vi "Make.vi"(8 "error in (no error)":errorcluster, 10 "Actor":string) -> (0 "error out":errorcluster, 3 "Test-Client out":refnum<class "Test-Client.lvclass">)   [LabVIEW 2020, in "Test-Client.lvlib" / "Test-Client.lvclass"]
uses:
  Test-Client.lvclass
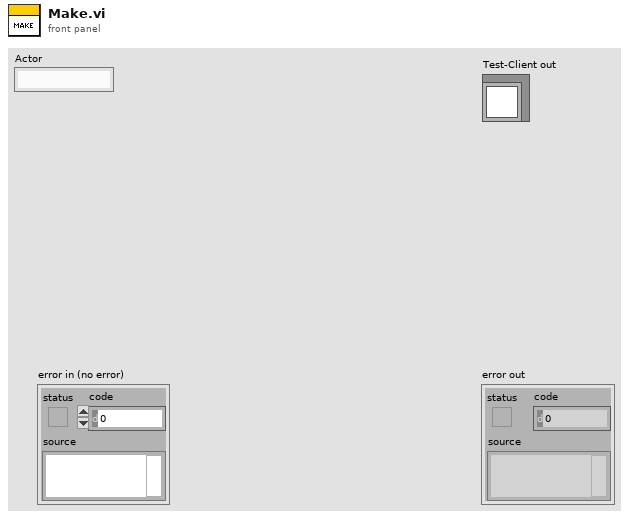
[diagram p1: front panel]
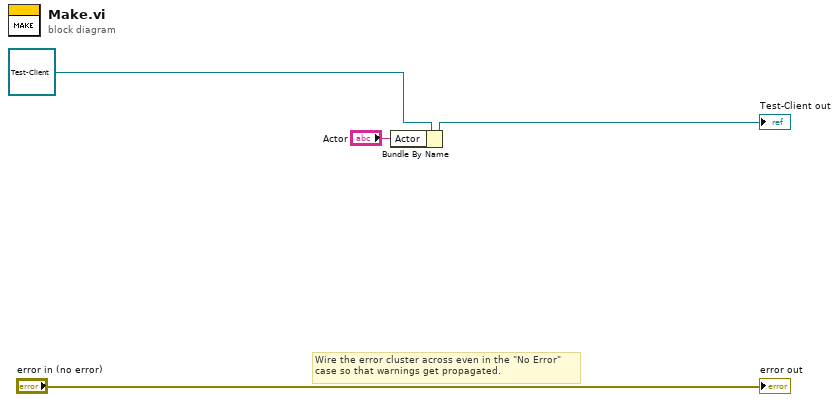
[diagram p0: block diagram]
diagram:
  # "Wire the error cluster across even in the \"No Error\"\ncase so that warnings get propagated."
  n1 = Bundle By Name(cluster=refnum<class "Test-Client.lvclass"> refnum ("Test-Client in"), "Actor"="Actor") -> (→"Test-Client out":refnum<class "Test-Client.lvclass">)
  "error out" <- "error in (no error)"
